vi "Expand Menu.vi"(8 "error in (no error)":errorcluster, 11 "MenuButton in":refnum<class "MenuButton.lvclass">) -> (0 "error out":errorcluster, 2 "Ending Bottom Position":u32, 3 "MenuButton out":refnum<class "MenuButton.lvclass">)   [LabVIEW 2017, in "MenuButtons.lvlib" / "MenuButton.lvclass"]
uses:
  MenuButton.lvclass
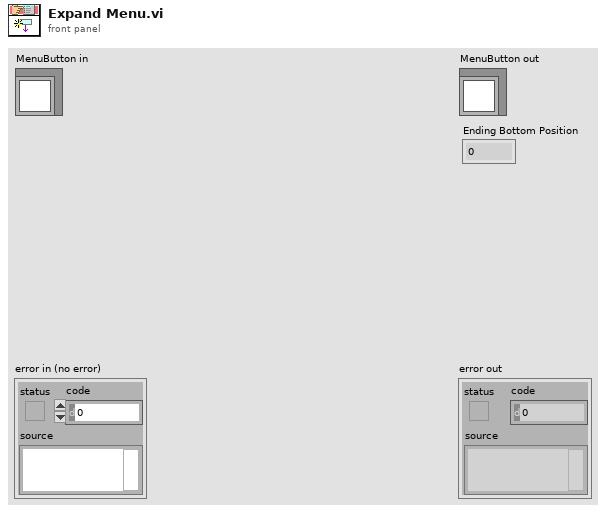
[diagram p1: front panel]
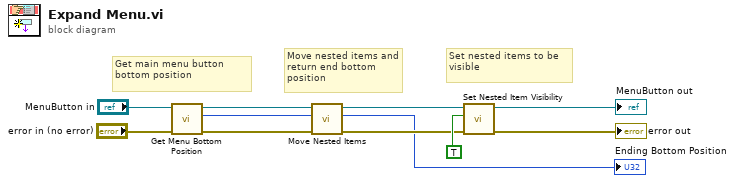
[diagram p0: block diagram]
diagram:
  # "Set nested items to be visible"
  # "Move nested items and return end bottom position"
  # "Get main menu button bottom position"
  n1 = call "Get Menu Bottom Position.vi"("error in (no error)"="error in (no error)", "MenuButton in"="MenuButton in") -> ("error out"=w5:errorcluster, "Menu Bottom Position"=w6:u32, "MenuButton out"=w7:refnum<class "MenuButton.lvclass">)  [unwired: 7 in]
  n2 = call "Move Nested Items.vi"("error in (no error)"=w5, "Starting Top Position"=w6, "MenuButton in"=w7) -> ("error out"=w4:errorcluster, "Ending Bottom Position"=→"Ending Bottom Position":u32, "MenuButton out"=w9:refnum<class "MenuButton.lvclass">)  [unwired: 6 in]
  n3 = call "Set Nested Item Visibility.vi"("error in (no error)"=w4, "Visible?"=TRUE, "MenuButton in"=w9) -> ("error out"=→"error out":errorcluster, "MenuButton out"=→"MenuButton out":refnum<class "MenuButton.lvclass">)  [unwired: 7 in]
